vi "TestEvents.vi"() -> ()   [LabVIEW 2017]
uses:
  Globals/globals.vi
panel:
  out "ExampleExpID":string
  out "ExpID":string
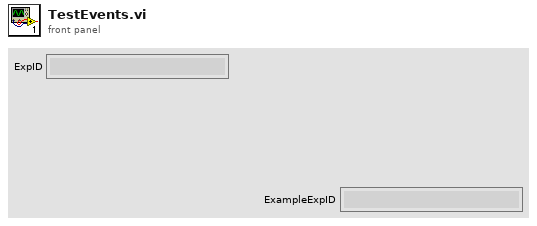
[diagram p1: front panel]
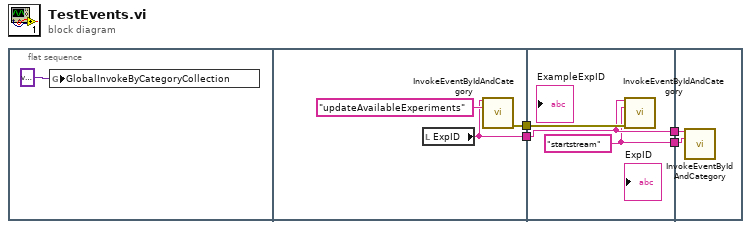
[diagram p0: block diagram]
diagram:
  n1 = flat-sequence {
    tunnel: [w7] -> w4
    tunnel: [w6] -> w3
    tunnel: w4 -> [w11]
    tunnel: w3 -> [w10]
    tunnel: [w10] -> w2
    tunnel: [w9] -> w1
    tunnel: w2 -> [w13]
    tunnel: w1 -> [w12]
    frame #0 {
      n2 = global write "globals.vi" "GlobalInvokeByCategoryCollection"(variant) -> ()
    }
    frame #1 {
      n3 = local read "ExpID"() -> (w6:string)
      n4 = call "InvokeEventByIdAndCategory.vi"("ID"=w6, "eventName"="updateAvailableExperiments" ("event data")) -> ("error out"=w7:errorcluster)  [unwired: 13 in]
    }
    frame #2 {
      w9 = "startstream" ("event data")
      n5 = call "InvokeEventByIdAndCategory.vi"("ID"=w10, "eventName"=w9, "error in (no error)"=w11) -> ()  [unwired: 12 in, 1 out]
    }
    frame #3 {
      n6 = call "InvokeEventByIdAndCategory.vi"("ID"=w13, "eventName"=w12) -> ()  [unwired: 13 in, 1 out]
    }
  }
